vi "Demo.vi"() -> ()   [LabVIEW 2011]
uses:
  MVCAMSDK.dll
panel:
  in  "切换到手动曝光模式":bool caption="软触发"
  in  "设置曝光时间（需要先设置为手动曝光模式）":bool caption="软触发"
  in  "曝光时间，单位微秒":dbl format="%#_6f"
  in  "切换到硬触发模式":bool caption="软触发"
  in  "切换到软触发模式":bool caption="软触发"
  in  "切换到连续模式":bool caption="软触发"
  in  "软触发":bool
  out "图像时间戳":u32 format="%_32g"
  out "Video":T1(plugin-control)
  in  "读取自定义数据":bool
  out "从相机中读出的字符串(32字节)":string
  in  "写入自定义数据":bool
  in  "要写入相机的字符串(32字节)":string
  in  "拍照":bool
  in  "显示相机参数面板":bool
  in  "Stop":bool
  in  "激活预览":bool=TRUE
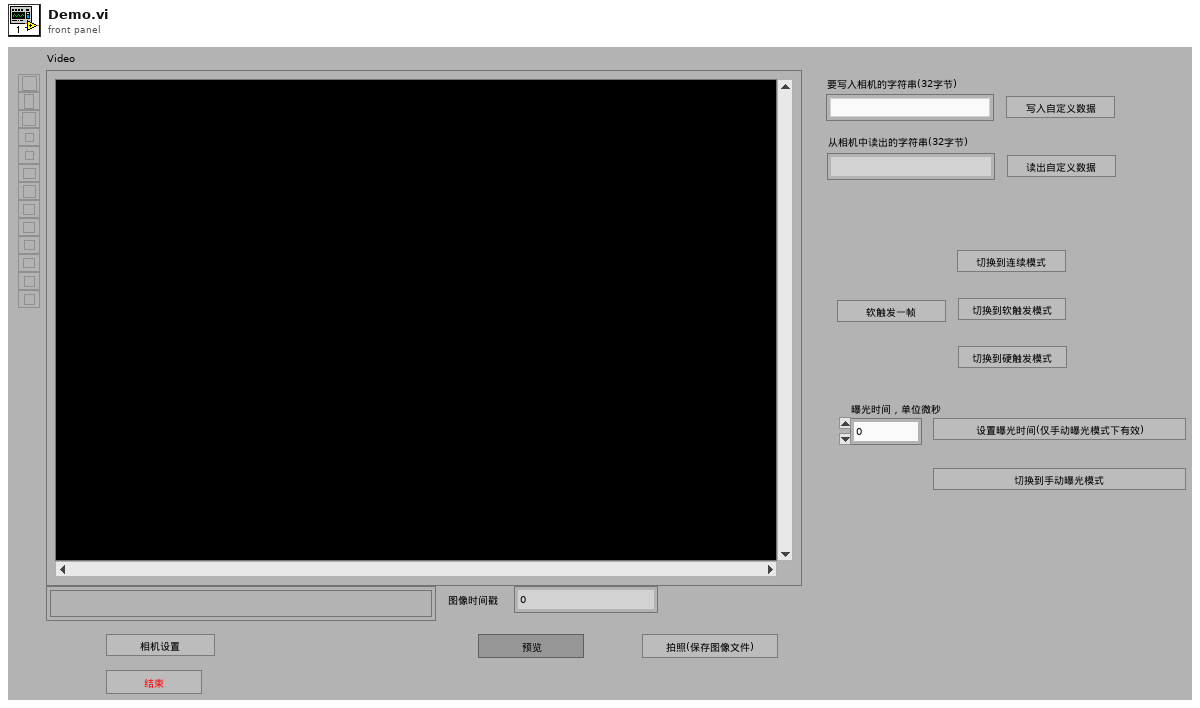
[diagram p1: front panel]
types:
  T1 = typedef "IMAQ Image.ctl" = refnum<image>
  T2 = typedef "Image Type" = u32
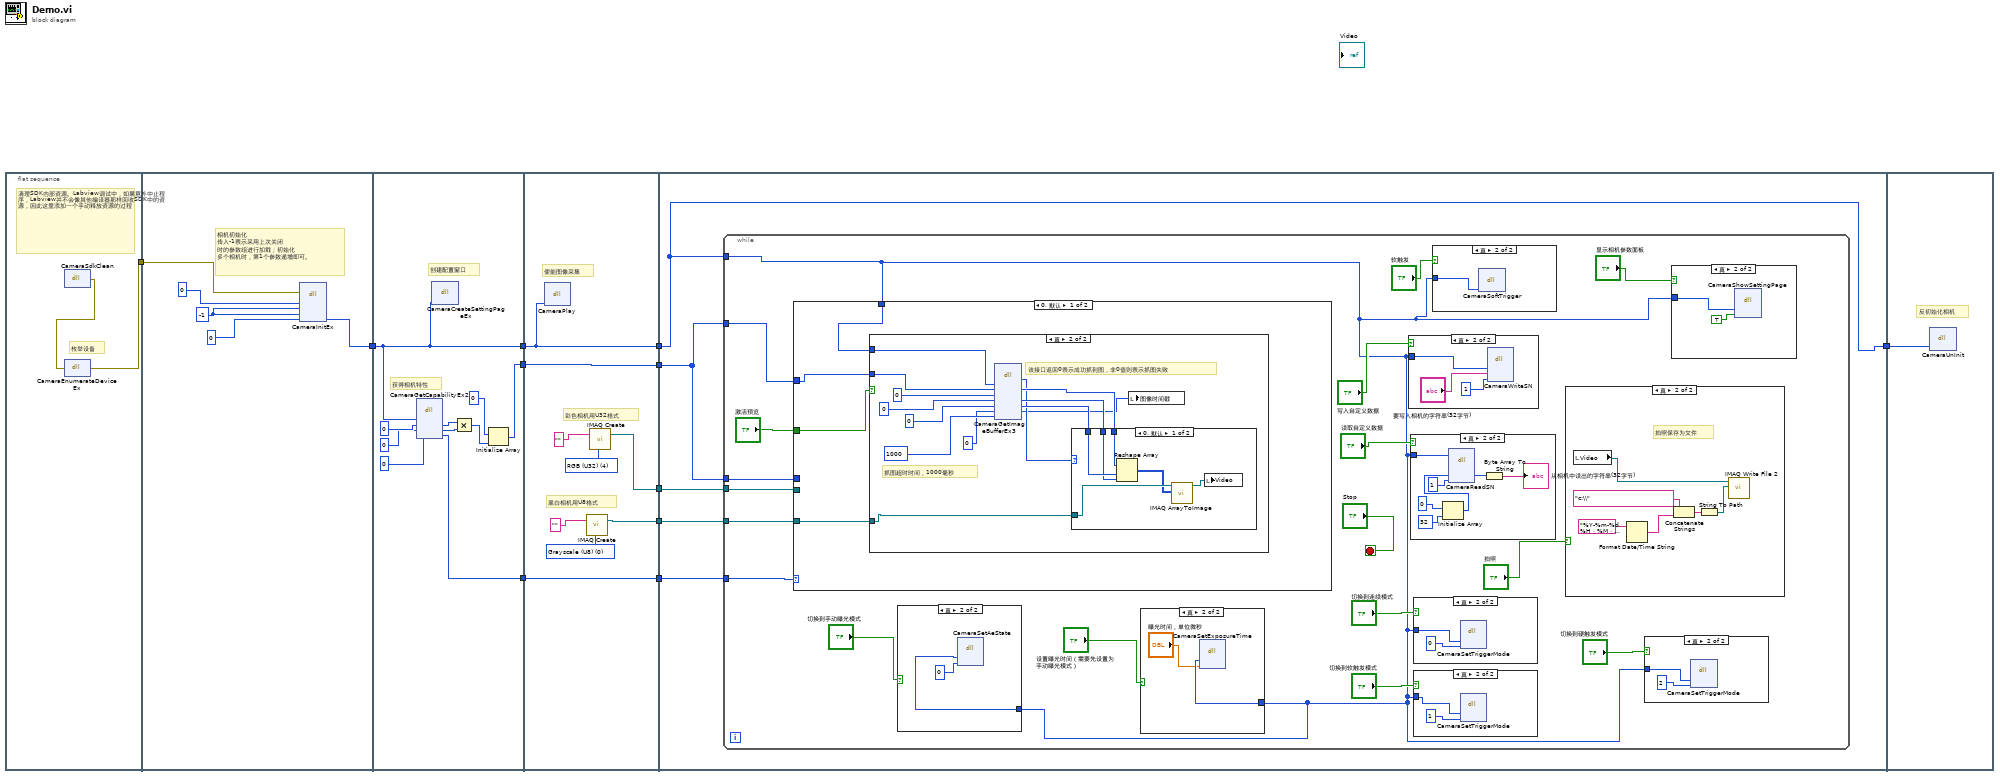
[diagram p0: block diagram]
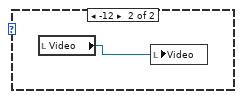
[diagram p11: hidden frame]
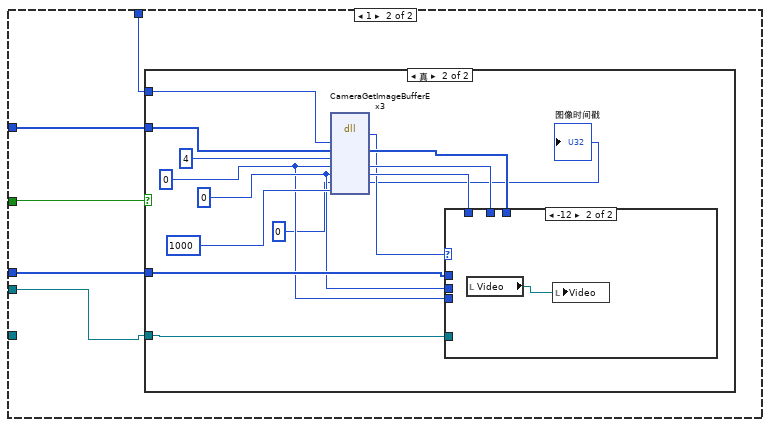
[diagram p12: hidden frame]
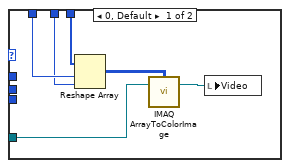
[diagram p14: hidden frame]
diagram:
  n1 = flat-sequence {
    tunnel: [w12] -> w1
    tunnel: [w15] -> w8
    tunnel: w1 -> [w14]
    tunnel: w8 -> [w25]
    tunnel: [w25] -> w7
    tunnel: [w26] -> w6
    tunnel: [w19] -> w4
    tunnel: w7 -> [w37]
    tunnel: [w37] -> w11
    tunnel: [w34] -> w9
    tunnel: w6 -> [w33]
    tunnel: [w33] -> w5
    tunnel: w4 -> [w32]
    tunnel: [w32] -> w3
    tunnel: [w29] -> w2
    tunnel: w11 -> [w40]
    tunnel: [w40] -> w10
    tunnel: w9 -> [w42]
    tunnel: w5 -> [w38]
    tunnel: w3 -> [w41]
    tunnel: w2 -> [w39]
    tunnel: w10 -> [w140]
    frame #0 {
      # "枚举设备"
      # "清理SDK内部资源。Labview调试中，如果意外中止程序，Labview并不会像其他编译器那样回收SDK中的资源，因此这里添加一个手动释放资源的过程"
      n2 = dll-call lib="MVCAMSDK.dll" fn="CameraSdkClean"() -> (error out=w13:errorcluster)  [unwired: 4 in, 1 out]
      n3 = dll-call lib="MVCAMSDK.dll" fn="CameraEnumerateDeviceEx"(error in=w13) -> (error out=w12:errorcluster)  [unwired: 3 in, 1 out]
    }
    frame #1 {
      w18 = -1
      # "相机初始化\n传入-1表示采用上次关闭\n时的参数组进行加载；初始化\n多个相机时，第1个参数递增即可。"
      n4 = dll-call lib="MVCAMSDK.dll" fn="CameraInitEx"(error in=w14, "相机索引值"=0, "参数加载方式"=w18, "要加载的参数组索引"=w18, "相机句柄"=0) -> ("相机句柄"=w15:i32)  [unwired: 6 in, 2 out]
    }
    frame #2 {
      # "获得相机特性"
      # "创建配置窗口"
      n5 = dll-call lib="MVCAMSDK.dll" fn="CameraGetCapabilityEx2"("相机句柄"=w25, "图像最大宽度"=0, "图像最大高度"=0, "是否是彩色相机(返回0:黑白;1:彩色)"=0) -> ("图像最大宽度"=w21:i32, "图像最大高度"=w20:i32, "是否是彩色相机(返回0:黑白;1:彩色)"=w19:i32)  [unwired: 5 in, 2 out]
      n6 = dll-call lib="MVCAMSDK.dll" fn="CameraCreateSettingPageEx"("相机句柄"=w25) -> ()  [unwired: 5 in, 2 out]
      n7 = Multiply(x=w21, y=w20) -> (x*y=w27:i32)
      n8 = Initialize Array(0, w27) -> (w26:i32[])
    }
    frame #3 {
      w31 = T2 0 items=["Grayscale (U8)", "Grayscale (I16)", "Grayscale (SGL)", "Complex (CSG)", "RGB (U32)", "HSL (U32)", "RGB (U64)", "Grayscale (U16)"] ("Image Type")
      w36 = T2 4 items=["Grayscale (U8)", "Grayscale (I16)", "Grayscale (SGL)", "Complex (CSG)", "RGB (U32)", "HSL (U32)", "RGB (U64)", "Grayscale (U16)"] ("Image Type")
      # "黑白相机用U8格式"
      # "彩色相机用U32格式"
      # "使能图像采集"
      n9 = dll-call lib="MVCAMSDK.dll" fn="CameraPlay"("相机句柄"=w37) -> ()  [unwired: 5 in, 2 out]
      n10 = call "IMAQ Create"("Image Name"="", "Image Type"=w31) -> ("New Image"=w29:T1)  [unwired: 3 in, 1 out]
      n11 = call "IMAQ Create"("Image Name"="", "Image Type"=w36) -> ("New Image"=w34:T1)  [unwired: 3 in, 1 out]
    }
    frame #4 {
      n12 = while {
        tunnel: w40 -> [w43]
        tunnel: w42 -> [w57]
        tunnel: w38 -> [w58]
        tunnel: w41 -> [w56]
        tunnel: w39 -> [w54]
        tunnel: w38 -> [w53]
        stop <- "Stop" stop-if-true
        n13 = case shown="0, 默认" w56 {
          tunnel: w58 -> [w83 w110]
          tunnel: w57 -> [_ w107]
          tunnel: w43 -> [w84 w109]
          tunnel: "激活预览" -> [w82 w108]
          tunnel: w54 -> [w85 _]
          tunnel: w53 -> [_ w106]
          frame 0, Default {
            n14 = case shown="真" w82 {
              tunnel: w84 -> [_ w98]
              tunnel: w83 -> [_ w89]
              tunnel: w85 -> [_ w88]
              frame False {
              }
              frame True {
                # "该接口返回0表示成功抓到图，非0值则表示抓图失败"
                # "抓图超时时间，1000毫秒"
                n15 = dll-call lib="MVCAMSDK.dll" fn="CameraGetImageBufferEx3"("相机句柄"=w98, "图像数据缓冲区"=w89, "图像输出格式(0:8位灰度;1:24位彩色;2:32位彩色，3：BGR24彩色 4：BGRA32位彩色)"=0, "图像宽度"=0, "图像高度"=0, "时间戳(单位为100微秒)"=0, "抓图超时时间(毫秒)"=1000) -> ("返回类型"=w90:i32, "图像数据缓冲区"=w93:u8[], "图像宽度"=w91:i32, "图像高度"=w92:i32, "时间戳(单位为100微秒)"=w86:u32)  [unwired: 6 in, 2 out]
                n16 = case shown="0, 默认" w90 {
                  tunnel: w93 -> [w104 _]
                  tunnel: w88 -> [w101 _]
                  tunnel: w92 -> [w103 _]
                  tunnel: w91 -> [w102 _]
                  frame 0, Default {
                    n17 = Reshape Array(w104, w103, w102) -> (w100:u8[][])
                    n18 = call "IMAQ ArrayToImage"("Image Pixels (U8)"=w100, "Image"=w101) -> ("Image Out"=w99:T1)  [unwired: 8 in, 1 out]
                    n19 = local write "Video"(w99) -> ()
                  }
                  frame -12 {
                    n20 = local read "Video"() -> (w105:T1)
                    n21 = local write "Video"(w105) -> ()
                  }
                }
                n22 = local write "图像时间戳"(w86) -> ()
              }
            }
          }
          frame 1 {
            n23 = case shown="真" w108 {
              tunnel: w109 -> [_ w124]
              tunnel: w107 -> [_ w117]
              tunnel: w110 -> [_ w116]
              tunnel: w106 -> [_ w115]
              frame False {
              }
              frame True {
                w113 = 0
                w114 = 0
                n24 = dll-call lib="MVCAMSDK.dll" fn="CameraGetImageBufferEx3"("相机句柄"=w124, "图像数据缓冲区"=w116, "图像输出格式(0:8位灰度;1:24位彩色;2:32位彩色)"=4, "图像宽度"=w113, "图像高度"=w114, "时间戳（单位为100微秒）"=0, "抓图超时时间(毫秒)"=1000) -> ("返回类型"=w118:i32, "图像数据缓冲区"=w121:u32[], "图像宽度"=w119:i32, "图像高度"=w120:i32, "时间戳（单位为100微秒）"=→"图像时间戳":u32)  [unwired: 6 in, 2 out]
                n25 = case shown="-12" w118 {
                  tunnel: w121 -> [w128 _]
                  tunnel: w117 -> [w127 _]
                  tunnel: w120 -> [w126 _]
                  tunnel: w119 -> [w125 _]
                  tunnel: w115 -> [_ _]
                  tunnel: w114 -> [_ _]
                  tunnel: w113 -> [_ _]
                  frame 0, Default {
                    n26 = Reshape Array(w128, w126, w125) -> (w129:u32[][])
                    n27 = call "IMAQ ArrayToColorImage"("Image Pixels (U32)"=w129, "Image"=w127) -> ("Image Out"=w130:T1)  [unwired: 3 in, 1 out]
                    n28 = local write "Video"(w130) -> ()
                  }
                  frame -12 {
                    n29 = local read "Video"() -> (w131:T1)
                    n30 = local write "Video"(w131) -> ()
                  }
                }
              }
            }
          }
        }
        n31 = case shown="真" "切换到手动曝光模式" {
          tunnel: w43 -> [_ w62]
          frame False {
          }
          frame True {
            n32 = dll-call lib="MVCAMSDK.dll" fn="CameraSetAeState"("相机句柄"=w62, "曝光模式(0手动，1自动)"=0) -> ()  [unwired: 6 in, 2 out]
          }
        }
        n33 = case shown="真" "设置曝光时间（需要先设置为手动曝光模式）" {
          tunnel: w43 -> [_ w64]
          frame False {
          }
          frame True {
            n34 = dll-call lib="MVCAMSDK.dll" fn="CameraSetExposureTime"("相机句柄"=w64, "曝光时间，单位微秒"="曝光时间，单位微秒") -> ()  [unwired: 6 in, 2 out]
          }
        }
        n35 = case shown="真" "写入自定义数据" {
          tunnel: w43 -> [_ w81]
          frame False {
          }
          frame True {
            n36 = dll-call lib="MVCAMSDK.dll" fn="CameraWriteSN"("相机句柄"=w81, "序列号(固定为32个字节)"="要写入相机的字符串(32字节)", "序列号级别，[0,1,2]对应3级序列号，其中0级为只读，1,2级可写"=1) -> ()  [unwired: 7 in, 2 out]
          }
        }
        n37 = case shown="真" "读取自定义数据" {
          tunnel: w43 -> [_ w78]
          frame False {
          }
          frame True {
            n38 = Initialize Array(0, 32) -> (w75:i32[])
            n39 = dll-call lib="MVCAMSDK.dll" fn="CameraReadSN"("相机句柄"=w78, "序列号"=w75, "序列号级别，[0,1,2],0级为只读，1,2级可写"=1) -> ("序列号"=w73:u8[])  [unwired: 6 in, 2 out]
            n40 = Byte Array To String(unsigned byte array=w73) -> (string=→"从相机中读出的字符串(32字节)":string)
          }
        }
        n41 = case shown="真" "切换到连续模式" {
          tunnel: w43 -> [_ w70]
          frame False {
          }
          frame True {
            n42 = dll-call lib="MVCAMSDK.dll" fn="CameraSetTriggerMode"("相机句柄"=w70, "模式"=0) -> ()  [unwired: 6 in, 2 out]
          }
        }
        n43 = case shown="真" "切换到软触发模式" {
          tunnel: w43 -> [_ w67]
          frame False {
          }
          frame True {
            n44 = dll-call lib="MVCAMSDK.dll" fn="CameraSetTriggerMode"("相机句柄"=w67, "模式"=1) -> ()  [unwired: 6 in, 2 out]
          }
        }
        n45 = case shown="真" "软触发" {
          tunnel: w43 -> [_ w71]
          frame False {
          }
          frame True {
            n46 = dll-call lib="MVCAMSDK.dll" fn="CameraSoftTrigger"("相机句柄"=w71) -> ()  [unwired: 5 in, 2 out]
          }
        }
        n47 = case shown="真" "拍照" {
          frame False {
          }
          frame True {
            # "拍照保存为文件"
            n48 = local read "Video"() -> (w132:T1)
            n49 = Format Date/Time String(time format string (%c)="%Y-%m-%d %H：%M：%S.bmp ") -> (date/time string=w136:string)  [unwired: 2 in]
            n50 = Concatenate Strings("c:\\", w136) -> (w133:string)
            n51 = String To Path(string=w133) -> (path=w135:path)
            n52 = call-poly "IMAQ Write File 2"("File Path"=w135, "Image"=w132) -> ()  [unwired: 8 in, 2 out]
          }
        }
        n53 = case shown="真" "切换到硬触发模式" {
          tunnel: w43 -> [_ w66]
          frame False {
          }
          frame True {
            n54 = dll-call lib="MVCAMSDK.dll" fn="CameraSetTriggerMode"("相机句柄"=w66, "模式"=2) -> ()  [unwired: 6 in, 2 out]
          }
        }
        n55 = case shown="真" "显示相机参数面板" {
          tunnel: w43 -> [_ w139]
          frame False {
          }
          frame True {
            n56 = dll-call lib="MVCAMSDK.dll" fn="CameraShowSettingPage"("相机句柄"=w139, "状态"=TRUE) -> ()  [unwired: 6 in, 2 out]
          }
        }
      }
    }
    frame #5 {
      # "反初始化相机"
      n57 = dll-call lib="MVCAMSDK.dll" fn="CameraUnInit"("相机句柄"=w140) -> ()  [unwired: 5 in, 2 out]
    }
  }
